vi "Delimit String.vi"(11 "Serial String":string) -> (2 "First Element":string, 3 "All Elements":string[](array[string]))   [LabVIEW 2015, in "RDS Serial Handler.lvlib"]
uses:
  RDS Serial Handler/RDS Serial Handler.lvlib
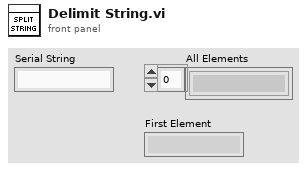
[diagram p1: front panel]
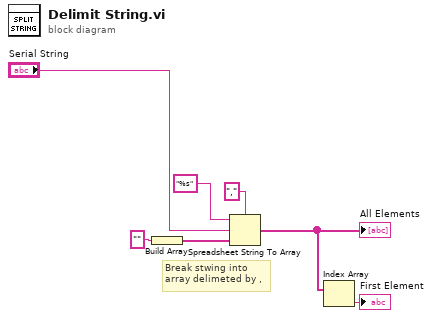
[diagram p0: block diagram]
diagram:
  # "Break stwing into\narray delimeted by ,"
  n1 = Build Array("") -> (w3:string[])
  n2 = Spreadsheet String To Array(delimiter (Tab)=",", format string="%s", spreadsheet string="Serial String", array type (2D Dbl)=w3) -> (array=w5:string[])
  "All Elements" <- w5
  n3 = Index Array(array=w5) -> (element=→"First Element":string)  [unwired: 1 in]
